vi "Globals.vi"() -> ()   [LabVIEW 2016]
panel:
  in  "Stop Search For Zero":bool
  in  "Stop Constant Query":bool
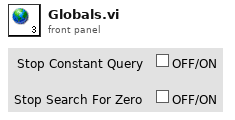
[diagram p1: front panel]
diagram:
